vi "Power, Conserve Sign.vi"(2 "Input":dbl, 3 "Power":i32) -> (0 "Output":dbl)   [LabVIEW 2012]
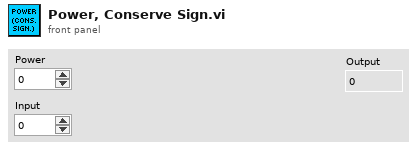
[diagram p1: front panel]
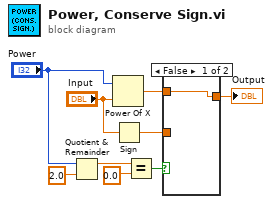
[diagram p0: block diagram]
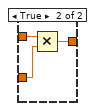
[diagram p2: hidden frame]
diagram:
  n1 = Quotient & Remainder(x="Power", y=2.0) -> (x-y*floor(x/y)=w8:dbl)  [unwired: 1 out]
  n2 = Power Of X(1:"Input", 2:"Power") -> (0:w3:dbl)
  n3 = Sign(1:"Input") -> (0:w4:dbl)
  n4 = Equal?(x=w8, y=0.0) -> (x = y?=w7:bool)
  n5 = case shown="False" w7 {
    tunnel: w4 -> [_ w13]
    tunnel: w3 -> [w10 w12]
    tunnel: [w10 w11] -> w2
    frame False {
    }
    frame True {
      n6 = Multiply(x=w12, y=w13) -> (x*y=w11:dbl)
    }
  }
  "Output" <- w2
